vi "configureTrigger_action.vi"(0 "HGF_Prosilica_GC655":refnum<class "HGF_Prosilica_GC655.lvclass">, 1 "Type":u32(ring) items=["External"=0, "RTSI"=1, "ISO In"=2, "Scaled Encoder"=5, "Software Trigger"=6], 2 "Line Number":u32, 3 "Frame timeout (ms)":u32=1000, 4 "Action":u32(ring) items=["Disabled", "Trigger start of acquisition", "Trigger start of each buffer list", "Trigger each buffer", "Trigger each line (linescan)", "Trigger end of acquisition"], 5 "error in (no error)":errorcluster, 6 "Activation":u32(ring) items=["Rising Edge", "Falling Edge", "AnyEdge", "LevelHigh", "LevelLow"], 7 "Delay":cluster{"Value":dbl, "Units":u32}={"Value"=0.0, "Units"=5} {"Units" items=["Scaled Encoder Counts"=4, "Milliseconds"=5]}, 8 "Mode":T1(ring), 9 "Skip trigger (linescan only)":u32) -> (14 "dup HGF_Prosilica_GC655":refnum<class "HGF_Prosilica_GC655.lvclass">, 19 "error out":errorcluster)   [LabVIEW 2014, in "HGF_IMAQ.lvlib" / "HGF_Prosilica_GC655.lvclass"]
doc: "Configures the trigger conditions for an acquisition. Use this VI before any acquisition VI to setup a triggered image acquisition."
uses:
  HGF_Prosilica_GC655.lvclass
  VisionTools/HGF_VisionTools/HGF_VisionTools.lvlib
  VisionTools/HGF_VisionTools/IMAQdx_setAttribute_Enum.vi
  HGF_Auxiliary/ErrorCode.ctl
  HGF_Auxiliary/HGF_Auxiliary.lvlib
  HGF_Auxiliary/Severity.ctl
  VisionTools/HGF_VisionTools/IMAQdx_setAttribute_Dbl.vi
  HGF_ImaqDx/HGF_ImaqDx.lvclass
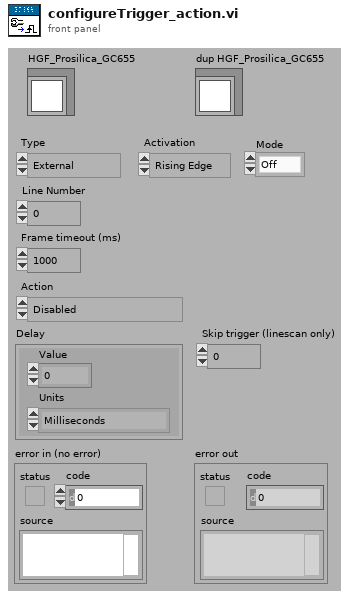
[diagram p1: front panel]
types:
  T1 = enum16{"Off", "Mode 0", "Mode 1", "Mode 2", "Mode 3", "Mode 4", "Mode 5"}
  T2 = typedef "HGF_Auxiliary.lvlib/Severity.ctl" = enum16{"Info", "Warning", "Fault", "Error", "Fatal"}
  T3 = typedef "HGF_Auxiliary.lvlib/ErrorCode.ctl" = enum32{"No error", "Function not supported.", "This VI is for friends only.", "Reference object aready exisits.", "Parameter out of range.", "Not a rendezvous.", "Invalid notifier reference.", "Invalid queue reference.", "Self-Test not supported.", "Reset not supported.", "IDN query not supported.", "Error query not supported.", "Incorrect addressee.", "Object already exists.", "No class name specified", "Driver not supported", "Attribute is not writable"}
  T4 = typedef "IMAQdx.ctl" = refnum<k21>
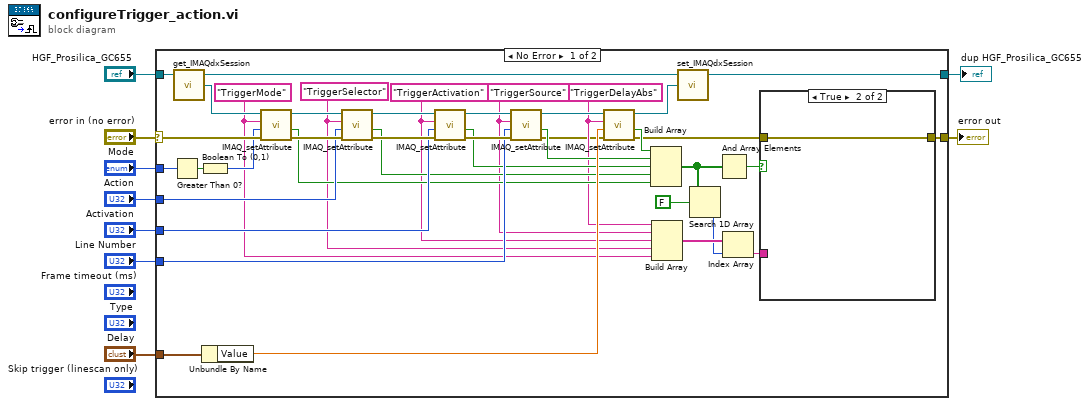
[diagram p0: block diagram]
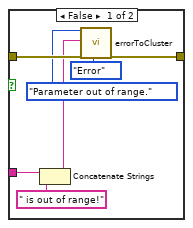
[diagram p2: hidden frame]
diagram:
  n1 = case shown="No Error" "error in (no error)" {
    selector: "error in (no error)" -> [w43 w58]
    tunnel: "HGF_Prosilica_GC655" -> [w32 w59]
    tunnel: [w42 w58] -> w7
    tunnel: [w28 w59] -> w8
    tunnel: "Activation" -> [w41 _]
    tunnel: "Mode" -> [w40 _]
    tunnel: "Line Number" -> [w37 _]
    tunnel: "Action" -> [w36 _]
    tunnel: "Delay" -> [w35 _]
    frame No Error {
      w16 = "TriggerDelayAbs" ("Attribute Name")
      w15 = "TriggerSource" ("Attribute Name")
      w14 = "TriggerActivation" ("Attribute Name")
      w12 = "TriggerMode" ("Attribute Name")
      w13 = "TriggerSelector" ("Attribute Name")
      n2 = Greater Than 0?(x=w40) -> (x > 0?=w39:bool)
      n3 = call "get_IMAQdxSession.vi"("HGF_ImaqDx in"=w32) -> ("IMAQdx Session"=w33:T4, "HGF_ImaqDx out"=w29:refnum<class "HGF_Prosilica_GC655.lvclass">)  [unwired: 2 in, 1 out]
      n4 = Boolean To (0,1)(Boolean=w39) -> (0, 1=w38:i16)
      n5 = Unbundle By Name(w35) -> ("Value"=w34:dbl)
      n6 = call-poly "IMAQ_setAttribute.vi"("error in (no error)"=w43, "Value (Enum)"=w38, "Attribute Name"=w12, "IMAQdx Session"=w33) -> ("error out"=w48:errorcluster, "In Range?"=w27:bool, "dup IMAQdx Session"=w49:T4)  [unwired: 1 in]
      n7 = call-poly "IMAQ_setAttribute.vi"("error in (no error)"=w48, "Value (Enum)"=w36, "Attribute Name"=w13, "IMAQdx Session"=w49) -> ("error out"=w46:errorcluster, "In Range?"=w26:bool, "dup IMAQdx Session"=w47:T4)  [unwired: 1 in]
      n8 = call-poly "IMAQ_setAttribute.vi"("error in (no error)"=w46, "Value (Enum)"=w41, "Attribute Name"=w14, "IMAQdx Session"=w47) -> ("error out"=w45:errorcluster, "In Range?"=w25:bool, "dup IMAQdx Session"=w44:T4)  [unwired: 1 in]
      n9 = call-poly "IMAQ_setAttribute.vi"("error in (no error)"=w45, "Value (Enum)"=w37, "Attribute Name"=w15, "IMAQdx Session"=w44) -> ("error out"=w11:errorcluster, "In Range?"=w24:bool, "dup IMAQdx Session"=w31:T4)  [unwired: 1 in]
      n10 = call-poly "IMAQ_setAttribute.vi"("error in (no error)"=w11, "Value (DBL)"=w34, "Attribute Name"=w16, "IMAQdx Session"=w31) -> ("error out"=w10:errorcluster, "In Range?"=w23:bool, "dup IMAQdx Session"=w30:T4)  [unwired: 1 in]
      n11 = Build Array(w23, w24, w25, w26, w27) -> (w21:bool[])
      n12 = Build Array(w16, w15, w14, w13, w12) -> (w19:string[])
      n13 = call "set_IMAQdxSession.vi"("IMAQdx Session"=w30, "HGF_ImaqDx in"=w29) -> ("HGF_ImaqDx out"=w28:refnum<class "HGF_Prosilica_GC655.lvclass">)  [unwired: 2 in, 1 out]
      n14 = Search 1D Array(1D array=w21, element=FALSE) -> (index of element=w18:i32)  [unwired: 1 in]
      n15 = And Array Elements(Boolean array=w21) -> (logical AND=w22:bool)
      n16 = Index Array(array=w19, index=w18) -> (element=w17:string)
      n17 = case shown="True" w22 {
        tunnel: w10 -> [w56 w57]
        tunnel: [w55 w57] -> w42
        tunnel: w17 -> [w52 _]
        frame False {
          n18 = Concatenate Strings(w52, " is out of range!" ("string")) -> (w51:string)
          n19 = call "errorToCluster.vi"("error code"=ErrorCode."Parameter out of range.", "error message (\"\")"=w51, "error in (no error)"=w56, "severity (Error)"=Severity."Error") -> ("error out"=w55:errorcluster)  [unwired: 15 in]
        }
        frame True {
        }
      }
    }
    frame Error {
    }
  }
  "error out" <- w7
  "dup HGF_Prosilica_GC655" <- w8
